vi "test variant to json var.vi"(8 "error in (no error)":errorcluster) -> (0 "error out":errorcluster)   [LabVIEW 2019, in "labview_json_tests.lvlib"]
uses:
  labview_json_tests.lvlib
  lib/Value.ctl
  lib/Value Type.ctl
  lib/labview_json.lvlib
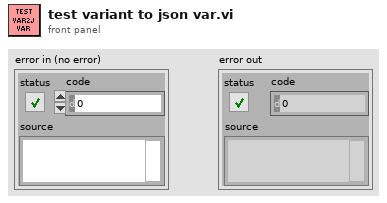
[diagram p1: front panel]
types:
  T1 = typedef "labview_json.lvlib/Value.ctl" = cluster{"Key":string, "Type":T2, "Value":variant}
  T2 = typedef "labview_json.lvlib/Value Type.ctl" = enum8{"NULL", "OBJECT", "ARRAY", "BOOL", "INT", "UINT", "FLOAT", "STRING"}
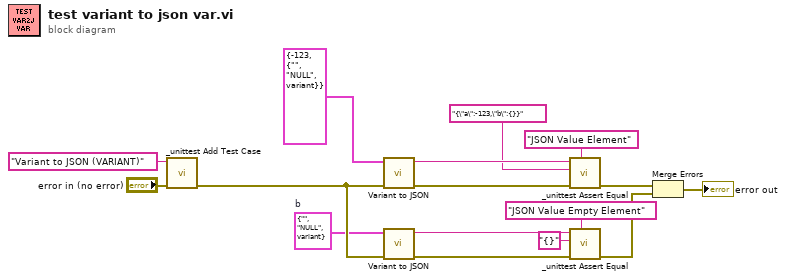
[diagram p0: block diagram]
diagram:
  w1 = T1 {"Key"="", "Type"=enum."NULL", "Value"=variant}  # b
  n1 = call "_unittest Add Test Case.vi"("error in (no error)"="error in (no error)", "Test Case"="Variant to JSON (VARIANT)") -> ("error out"=w4:errorcluster)  [unwired: 9 in]
  n2 = call "Variant to JSON.vi"("error in (no error)"=w4, "Variant in"=cluster{"a":i32, "b":T1} {"a"=-123, "b"={"Key"="", "Type"=enum."NULL", "Value"=variant}} ("Cluster")) -> ("error out"=w11:errorcluster, "JSON"=w10:string)  [unwired: 8 in]
  n3 = call "Variant to JSON.vi"("error in (no error)"=w4, "Variant in"=w1) -> ("error out"=w6:errorcluster, "JSON"=w7:string)  [unwired: 8 in]
  n4 = call "_unittest Assert Equal.vi"("Message"="JSON Value Element", "error in (no error)"=w11, "Expected Value"="{\"a\":-123,\"b\":{}}", "Actual Value"=w10) -> ("error out"=w14:errorcluster)  [unwired: 7 in]
  n5 = call "_unittest Assert Equal.vi"("Message"="JSON Value Empty Element", "error in (no error)"=w6, "Expected Value"="{}", "Actual Value"=w7) -> ("error out"=w3:errorcluster)  [unwired: 7 in]
  n6 = Merge Errors(w14, w3) -> (→"error out":errorcluster)
